vi "Teleop.vi"(10 "Match Info":T1={"Autonomous Elapsed Seconds"=0.0, "TeleOp Elapsed Seconds"=0.0, "Disabled Elapsed Seconds"=0.0, "Visited Autonomous"=FALSE, "Visited TeleOp"=FALSE, "Visited Disabled"=FALSE, "Autonomous Settings"={"Autonomous Style"=enum."Independent", "VI Refnum"=refnum}}, 11 "Call Context":T2) -> ()   [LabVIEW 2015]
doc: "This VI is called for each TeleOp packet received from the DS where the robot is not disabled. It is often used to read from the joysticks and update I/O or to update setpoints for timed control loops. It should complete and return within 20 milliseconds or it may miss DS packets."
uses:
  <vilib>/Rock Robotics/WPI/DriverStation/WPI_DriverStationDerivedRobotMode.ctl
  <vilib>/Rock Robotics/WPI/DriverStation/WPI_DriverStationMatch Info.ctl
  <vilib>/Rock Robotics/WPI/Utilities/WPI_GetSetVariantRefNum.vi
  <vilib>/Rock Robotics/Network Tables/NT Write Boolean Array.vi
  <vilib>/Rock Robotics/Network Tables/NT Write Numeric Array.vi
  <vilib>/Rock Robotics/Network Tables/NT Read Boolean.vi
  <vilib>/Rock Robotics/Network Tables/NT Read Number.vi
  <vilib>/Rock Robotics/Network Tables/NT Write Number.vi
  <vilib>/Rock Robotics/Network Tables/NT Write Boolean.vi
panel:
  out "Sample Slider 0":dbl(slide) scale=0.0..5.0
  out "Sample Boolean 1":bool
  out "Sample Boolean 0":bool
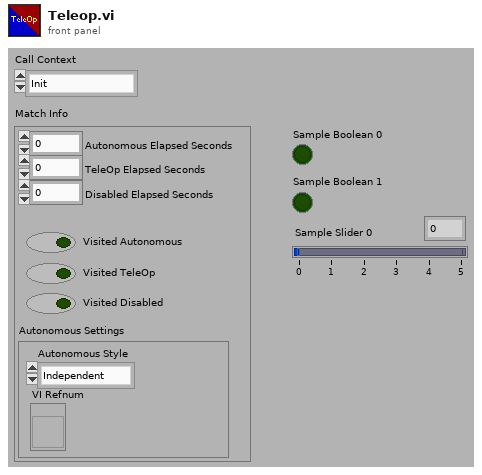
[diagram p1: front panel]
types:
  T1 = typedef "WPI_DriverStationMatch Info.ctl" = cluster{"Autonomous Elapsed Seconds":dbl, "TeleOp Elapsed Seconds":dbl, "Disabled Elapsed Seconds":dbl, "Visited Autonomous":bool, "Visited TeleOp":bool, "Visited Disabled":bool, "Autonomous Settings":cluster{"Autonomous Style":enum16{"Iterative", "Independent"}, "VI Refnum":refnum<vi>}}
  T2 = typedef "WPI_DriverStationDerivedRobotMode.ctl" = enum16{"Init", "Execute", "Stop"}
  T3 = typedef "WPI_DriverStationAllianceInfo.ctl" = enum16{"Red", "Blue", "Invalid"}
  T4 = typedef "WPI_GyroDevRef.ctl" = cluster{"DevStatus":errorcluster, "Analog Channel":T5, "Offset":dbl, "Gain (VoltsPerDegree/Second)":dbl, "Gyro Type":enum16{"Analog", "XRS450"}, "Handle":i32, "SPI Bus":T6, "Device Found":bool, "Sample Rate":dbl, "Calibrate On Open":bool}
  T5 = typedef "FPGA_AIChannel.ctl" = enum8{"AI 0", "AI 1", "AI 2", "AI 3", "AI MXP 0", "AI MXP 1", "AI MXP 2", "AI MXP 3", "Invalid"}
  T6 = typedef "spi_bus.ctl" = enum16{"SPI On-Board, CS0", "SPI On-Board, CS1", "SPI On-Board, CS2", "SPI On-Board, CS3", "SPI MXP", "Invalid"}
  T7 = typedef "WPI_AccelerometerDevRef.ctl" = cluster{"DevStatus":errorcluster, "Scaling":T8, "Analog Channels":T9, "I2C Bus":T10, "SPI Bus":T6, "Accel Range":T11, "ADXL Axes":T12, "Handle":i32, "Device Address":u8, "Accel Type":enum16{"Analog", "ADXL345 I2C", "ADXL345 SPI", "Internal", "ADXL362 SPI"}}
  T8 = typedef "WPI_AccelerometerScaling.ctl" = cluster{"Gain (VoltsPerG)":dbl, "Center Voltage":dbl}
  T9 = typedef "WPI_AccelerometerAnalogChannels.ctl" = cluster{"X-Axis":T5, "Y-Axis":T5, "Z-Axis":T5}
  T10 = typedef "i2c_bus.ctl" = enum16{"I2C On-Board", "I2C MXP", "Invalid"}
  T11 = typedef "ADXL345 Range.ctl" = u8
  T12 = typedef "WPI_AccelerometerADXL345 Axes.ctl" = cluster{"X-Axis":bool, "Y-Axis":bool, "Z-Axis":bool}
  T13 = typedef "WPI_JoystickDevRef.ctl" = cluster{"Device":T14}
  T14 = typedef "WPI_JoystickDeviceEnum.ctl" = enum16{"USB 0", "USB 1", "USB 2", "USB 3", "USB 4", "USB 5"}
  T15 = cluster{"X-Axis":dbl, "Y-Axis":dbl, "Z-Axis":dbl}
  T16 = cluster{"Axes[0]":dbl, "Axes[1]":dbl, "Axes[2]":dbl, "Axes[3]":dbl, "Axes[4]":dbl, "Axes[5]":dbl, "Axes[6]":dbl, "Axes[7]":dbl, "Axes[8]":dbl}
  T17 = cluster{"Buttons[0]":bool, "Buttons[1]":bool, "Buttons[2]":bool, "Buttons[3]":bool, "Buttons[4]":bool, "Buttons[5]":bool, "Buttons[6]":bool, "Buttons[7]":bool, "Buttons[8]":bool}
  T18 = typedef "WPI_RobotDriveDevRef.ctl" = cluster{"DevStatus":errorcluster, "Motors[]":T19[], "Square Inputs":bool, "Max Output":dbl}
  T19 = typedef "WPI_MotorControlDeviceRef.ctl" = cluster{"DeviceStatus":errorcluster, "Type":T20, "PWM":cluster{"PWM Channel":T21, "DeadBand":T22}, "CAN":cluster{"Device Number":u8, "Control Mode":T23, "Semaphore":T24, "Max Vout":dbl, "TalonSRX Control Mode":T25}, "Invert":bool}
  T20 = typedef "WPI_MotorControlType.ctl" = enum16{"PWM", "CAN", "CANTalonSRX"}
  T21 = typedef "FPGA_DIOPWMChannel.ctl" = enum8{"PWM 0", "PWM 1", "PWM 2", "PWM 3", "PWM 4", "PWM 5", "PWM 6", "PWM 7", "PWM 8", "PWM 9", "PWM MXP 0", "PWM MXP 1", "PWM MXP 2", "PWM MXP 3", "PWM MXP 4", "PWM MXP 5", "PWM MXP 6", "PWM MXP 7", "PWM MXP 8", "PWM MXP 9", "Invalid"}
  T22 = typedef "WPI_PWMDeadband.ctl" = cluster{"Name":string, "maxPositivePwm":i32, "minPositivePwm":i32, "centerPwm":i32, "maxNegativePwm":i32, "minNegativePwm":i32, "angularRange":u16}
  T23 = typedef "WPI_CANJaguar_ControlMode.ctl" = enum8{"Percent VBus", "Current", "Speed", "Position", "Voltage"}
  T24 = typedef "Semaphore RefNum" = refnum<k1>
  T25 = typedef "WPI_CANTalonSRX_APIControlMode.ctl" = enum8{"Percent VBus", "Speed", "Position", "Slave", "Unchanged / Invalid", "Voltage Compensation", "Current", "Motion Profile"}
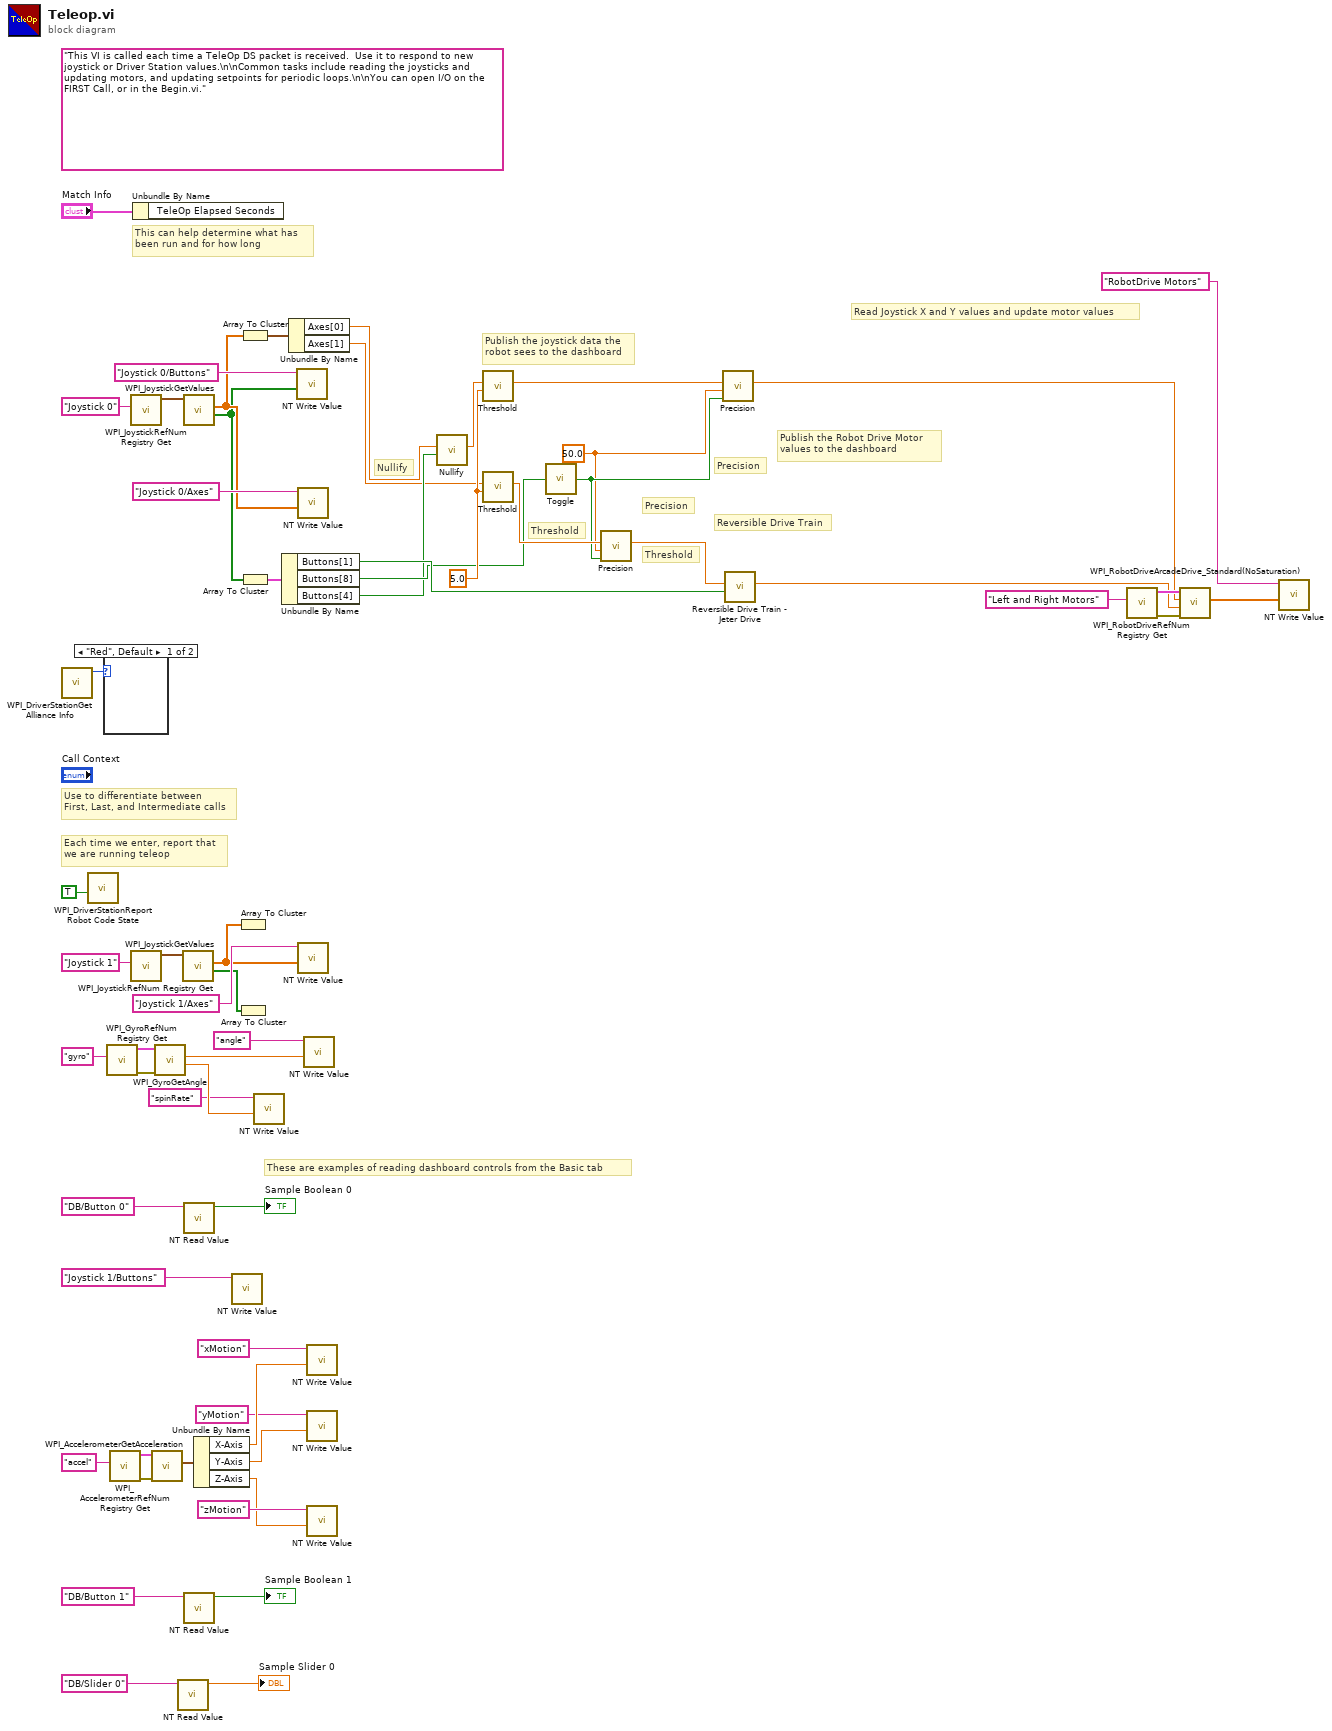
[diagram p0: block diagram]
diagram:
  w8 = 50.0 ("Percent Power")
  w14 = 5.0 ("Threshold")
  (unwired) "This VI is called each time a TeleOp DS packet is received.  Use it to respond to new joystick or Driver Station values.\n\nCommon tasks include reading the joysticks and updating motors, and updating setpoints for periodic loops.\n\nYou can open I/O on the FIRST Call, or in the Begin.vi."
  # "Nullify"
  # "Precision"
  # "Precision"
  # "Reversible Drive Train"
  # "Threshold"
  # "Threshold"
  # "These are examples of reading dashboard controls from the Basic tab"
  # "Publish the Robot Drive Motor\nvalues to the dashboard"
  # "Publish the joystick data the\nrobot sees to the dashboard"
  # "Each time we enter, report that\nwe are running teleop"
  # "Use to differentiate between\nFirst, Last, and Intermediate calls"
  # "This can help determine what has\nbeen run and for how long"
  # "Read Joystick X and Y values and update motor values"
  n1 = call <vilib>:"WPI_DriverStationGet Alliance Info.vi"() -> ("Alliance"=w16:T3)  [unwired: 11 out]
  n2 = call <vilib>:"WPI_DriverStationReport Robot Code State.vi"("TeleOp"=TRUE ("Autonomous")) -> ()  [unwired: 10 in, 1 out]
  n3 = case shown="\"Red\", Default" w16 {
    frame "Red", Default {
    }
    frame "Blue" {
    }
  }
  n4 = call <vilib>:"WPI_GyroRefNum Registry Get.vi"("refnum name"="gyro") -> ("error out"=w42:errorcluster, "GyroDevRef"=w43:T4)  [unwired: 9 in]
  n5 = call <vilib>:"WPI_AccelerometerRefNum Registry Get.vi"("refnum name"="accel") -> ("error out"=w41:errorcluster, "AccelerometerDevRef"=w40:T7)  [unwired: 9 in]
  n6 = call <vilib>:"WPI_JoystickRefNum Registry Get.vi"("refnum name"="Joystick 0") -> ("JoystickDevRef"=w55:T13)  [unwired: 1 in, 9 out]
  n7 = call <vilib>:"WPI_JoystickRefNum Registry Get.vi"("refnum name"="Joystick 1") -> ("JoystickDevRef"=w25:T13)  [unwired: 1 in, 9 out]
  n8 = Unbundle By Name("Match Info") -> ()  [unwired: 1 out]
  n9 = call <vilib>:"WPI_AccelerometerGetAcceleration.vi"("error in"=w41, "AccelerometerDevRef"=w40) -> ("Accelerations"=w35:T15)  [unwired: 7 in, 2 out]
  n10 = call <vilib>:"WPI_GyroGetAngle.vi"("error in"=w42, "GyroDevRef"=w43) -> ("Angular Rate"=w18:dbl, "Angle"=w37:dbl)  [unwired: 5 in, 3 out]
  n11 = call-poly <vilib>:"NT Read Value.vi"("Name"="DB/Slider 0" ("refnum name")) -> ("Numeric"=→"Sample Slider 0":dbl)  [unwired: 9 in, 1 out]
  n12 = call <vilib>:"WPI_JoystickGetValues.vi"("JoystickDevRef"=w25) -> ("Buttons"=w21:bool[], "Axes"=w22:dbl[])  [unwired: 6 in, 3 out]
  n13 = call <vilib>:"WPI_JoystickGetValues.vi"("JoystickDevRef"=w55) -> ("Buttons"=w29:bool[], "Axes"=w30:dbl[])  [unwired: 6 in, 3 out]
  n14 = call-poly <vilib>:"NT Read Value.vi"("Name"="DB/Button 0" ("refnum name")) -> ("Boolean"=→"Sample Boolean 0":bool)  [unwired: 9 in, 1 out]
  n15 = call-poly <vilib>:"NT Read Value.vi"("Name"="DB/Button 1" ("refnum name")) -> ("Boolean"=→"Sample Boolean 1":bool)  [unwired: 9 in, 1 out]
  n16 = Unbundle By Name(w35) -> ("X-Axis"=w34:dbl, "Y-Axis"=w32:dbl, "Z-Axis"=w19:dbl)
  n17 = call-poly <vilib>:"NT Write Value.vi"("Name"="Joystick 1/Buttons") -> ()  [unwired: 10 in, 1 out]
  n18 = Array To Cluster(array=w22) -> ()  [unwired: 1 out]
  n19 = Array To Cluster(array=w21) -> ()  [unwired: 1 out]
  n20 = Array To Cluster(array=w30) -> (cluster=w28:T16)
  n21 = Array To Cluster(array=w29) -> (cluster=w27:T17)
  n22 = call-poly <vilib>:"NT Write Value.vi"("Numeric"=w18, "Name"="spinRate") -> ()  [unwired: 9 in, 1 out]
  n23 = Unbundle By Name(w27) -> ("Buttons[1]"=w15:bool, "Buttons[8]"=w11:bool, "Buttons[4]"=w6:bool)
  n24 = Unbundle By Name(w28) -> ("Axes[0]"=w5:dbl, "Axes[1]"=w4:dbl)
  n25 = call-poly <vilib>:"NT Write Value.vi"("Boolean Array"=w29, "Name"="Joystick 0/Buttons") -> ()  [unwired: 9 in, 1 out]
  n26 = call-poly <vilib>:"NT Write Value.vi"("Numeric Array"=w30, "Name"="Joystick 0/Axes") -> ()  [unwired: 9 in, 1 out]
  n27 = call-poly <vilib>:"NT Write Value.vi"("Numeric Array"=w22, "Name"="Joystick 1/Axes") -> ()  [unwired: 9 in, 1 out]
  n28 = call-poly <vilib>:"NT Write Value.vi"("Numeric"=w37, "Name"="angle") -> ()  [unwired: 9 in, 1 out]
  n29 = call-poly <vilib>:"NT Write Value.vi"("Numeric"=w34, "Name"="xMotion") -> ()  [unwired: 9 in, 1 out]
  n30 = call-poly <vilib>:"NT Write Value.vi"("Numeric"=w32, "Name"="yMotion") -> ()  [unwired: 9 in, 1 out]
  n31 = call-poly <vilib>:"NT Write Value.vi"("Numeric"=w19, "Name"="zMotion") -> ()  [unwired: 9 in, 1 out]
  n32 = call "Nullify.vi"("Null?"=w6, "Number In"=w5) -> ("Number Out"=w7:dbl)  [unwired: 9 in]
  n33 = call "Threshold.vi"("Threshold Percent"=w14, "Number In"=w7) -> ("Number Out"=w10:dbl)  [unwired: 9 in]
  n34 = call "Threshold.vi"("Threshold Percent"=w14, "Number In"=w4) -> ("Number Out"=w12:dbl)  [unwired: 9 in]
  n35 = call "Toggle.vi"("Input"=w11) -> ("Output"=w9:bool)
  n36 = call "Precision.vi"("Precise?"=w9, "Percent Power"=w8, "Number In"=w12) -> ("Number Out"=w13:dbl)  [unwired: 8 in]
  n37 = call "Precision.vi"("Precise?"=w9, "Percent Power"=w8, "Number In"=w10) -> ("Number Out"=w2:dbl)  [unwired: 8 in]
  n38 = call "Reversible Drive Train - Jeter Drive.vi"("Flip"=w15, "Number In"=w13) -> ("Number Out"=w3:dbl)  [unwired: 9 in]
  n39 = call <vilib>:"WPI_RobotDriveRefNum Registry Get.vi"("refnum name"="Left and Right Motors") -> ("error out"=w1:errorcluster, "RobotDriveDevRef"=w57:T18)  [unwired: 1 in, 8 out]
  n40 = call <vilib>:"WPI_RobotDriveArcadeDrive_Standard(NoSaturation).vi"("error in (no error)"=w1, "Y axis value"=w3, "X axis value"=w2, "RobotDriveDevRef"=w57) -> ("Motor Values"=w45:dbl[])  [unwired: 7 out]
  n41 = call-poly <vilib>:"NT Write Value.vi"("Numeric Array"=w45, "Name"="RobotDrive Motors") -> ()  [unwired: 9 in, 1 out]
